vi "Read Position.vi"(8 "error in (no error)":errorcluster, 11 "Contestant in":refnum<class "Contestant.lvclass">) -> (0 "error out":errorcluster, 2 "Position":i32, 3 "Contestant out":refnum<class "Contestant.lvclass">)   [LabVIEW 2024, in "Contestant.lvlib" / "Contestant.lvclass"]
uses:
  Contestant.lvclass
  Contestant.lvclass/Contestant.ctl
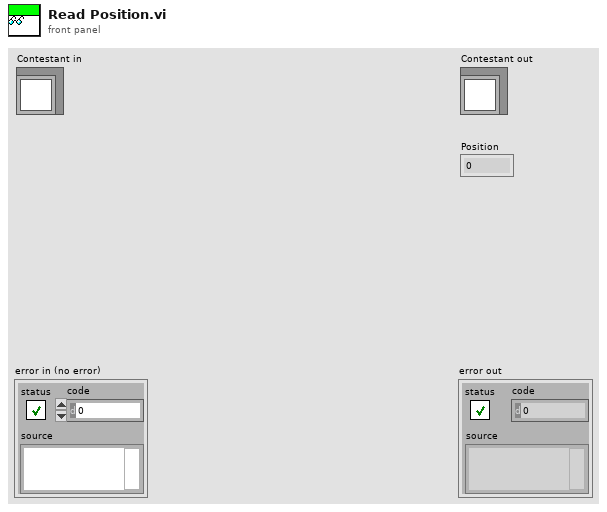
[diagram p1: front panel]
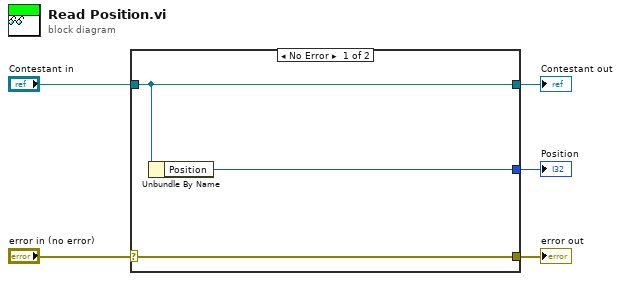
[diagram p0: block diagram]
diagram:
  n1 = case shown="No Error" "error in (no error)" {
    selector: "error in (no error)" -> [w8 w9]
    tunnel: [w8 w9] -> w4
    tunnel: [w7 w10] -> w2
    tunnel: "Contestant in" -> [w7 w10]
    tunnel: [w6 _] -> w1
    frame No Error {
      n2 = Unbundle By Name(w7) -> ("Position"=w6:i32)
    }
    frame Error {
    }
  }
  "error out" <- w4
  "Contestant out" <- w2
  "Position" <- w1
